vi "ShutterControls.vi"() -> ()   [LabVIEW 2019]
panel:
  in  "Numeric":dbl min=0.0 max=5.0
  in  "Button":bool
  in  "Stop":bool
  in  "Open Shutter":bool
  in  "Pict Ring":u16(ring)
  in  "LaserStatus":bool
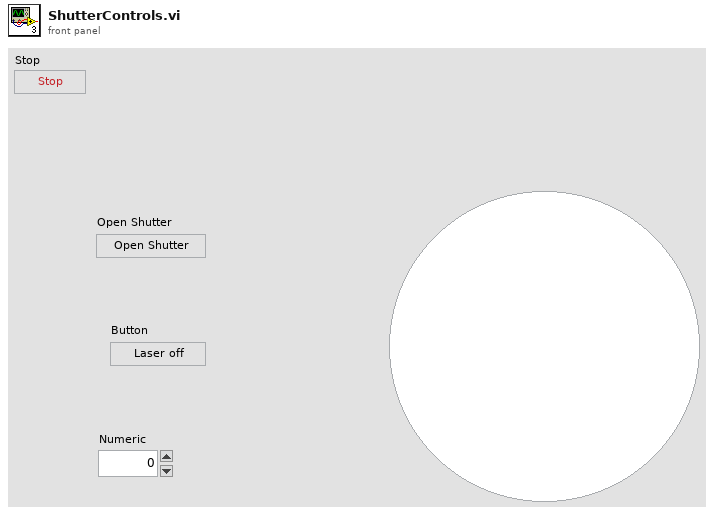
[diagram p1: front panel]
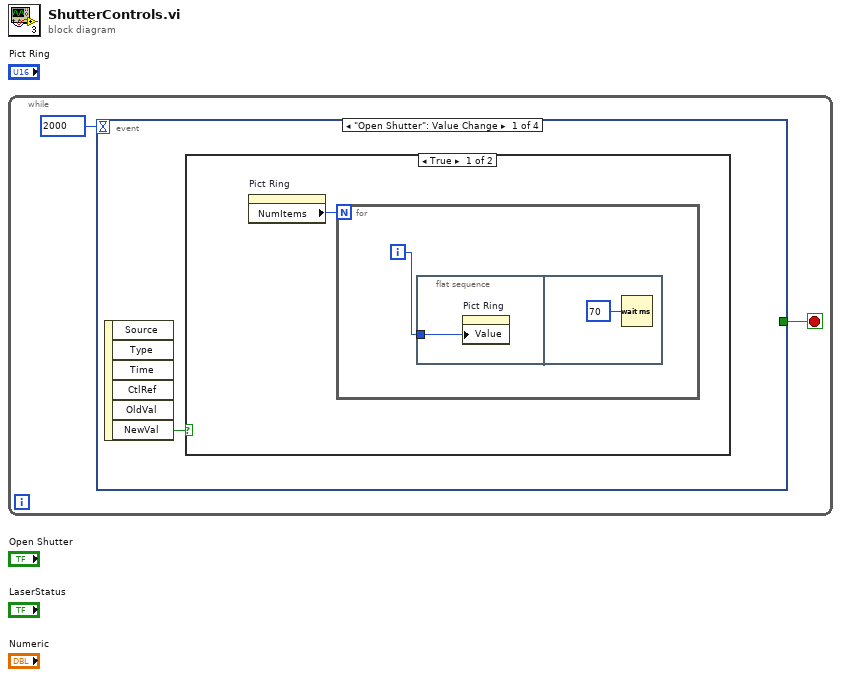
[diagram p0: block diagram]
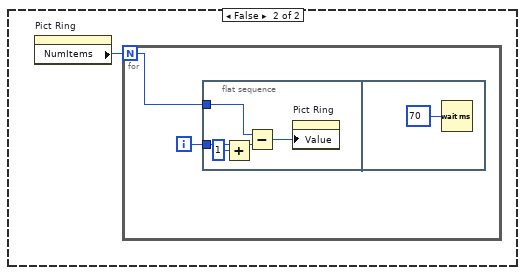
[diagram p2: hidden frame]
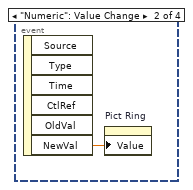
[diagram p3: hidden frame]
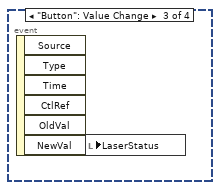
[diagram p4: hidden frame]
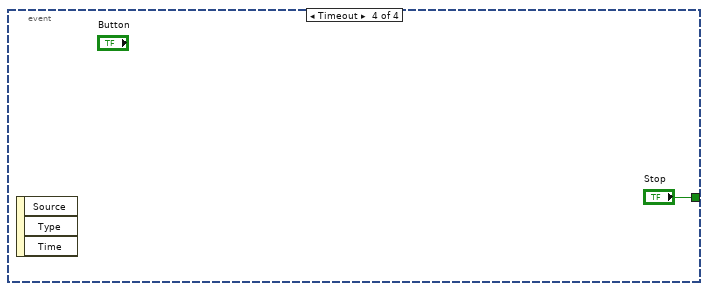
[diagram p5: hidden frame]
diagram:
  n1 = while {
    stop <- w1 stop-if-true
    n2 = event shown="[0] \"Open Shutter\": Value Change" {
      selector: _ -> [_ _ _ _]
      dyn-events: _ -> [_ _ _ _]
      timeout: 2000 -> [_ _ _ _]
      tunnel: [_ _ _ "Stop"] -> w1
      event "Open Shutter": Value Change {
        n3 = event-data() -> ("NewVal"=w3:bool)  [unwired: 1 in, 5 out]
        n4 = case shown="True" w3 {
          frame True {
            n5 = property on="Pict Ring" class="Ring (strict)"() -> ("NumItems"=w4:u32)  [unwired: 2 in, 2 out]
            n6 = for {
              N: w4 -> [_]
              i -> [w5]
              n7 = flat-sequence {
                tunnel: w5 -> [w6]
                frame #0 {
                  n8 = property on="Pict Ring" class="Ring (strict)"("Value"=w6) -> ()  [unwired: 2 in, 2 out]
                }
                frame #1 {
                  n9 = Wait (ms)(milliseconds to wait=u32 70) -> ()  [unwired: 1 out]
                }
              }
            }
          }
          frame False {
            n10 = property on="Pict Ring" class="Ring (strict)"() -> ("NumItems"=w8:u32)  [unwired: 2 in, 2 out]
            n11 = for {
              N: w8 -> [w10]
              i -> [w9]
              n12 = flat-sequence {
                tunnel: w9 -> [w12]
                tunnel: w10 -> [w15]
                frame #0 {
                  n13 = Add(x=w12, y=1) -> (x+y=w13:i32)
                  n14 = Subtract(x=w15, y=w13) -> (x-y=w14:i32)
                  n15 = property on="Pict Ring" class="Ring (strict)"("Value"=w14) -> ()  [unwired: 2 in, 2 out]
                }
                frame #1 {
                  n16 = Wait (ms)(milliseconds to wait=u32 70) -> ()  [unwired: 1 out]
                }
              }
            }
          }
        }
      }
      event "Numeric": Value Change {
        n17 = event-data() -> ("NewVal"=w17:dbl)  [unwired: 1 in, 5 out]
        n18 = property on="Pict Ring" class="Ring (strict)"("Value"=w17) -> ()  [unwired: 2 in, 2 out]
      }
      event "Button": Value Change {
        n19 = event-data() -> ("NewVal"=w18:bool)  [unwired: 1 in, 5 out]
        n20 = local write "LaserStatus"(w18) -> ()
      }
      event Timeout {
        n21 = event-data() -> ()  [unwired: 1 in, 3 out]
      }
    }
  }
